vi "Simulator SNA Measure.vi"(8 "error in (no error)":errorcluster, 10 "SP Stimulus":T5={"Use Instrument Settings"=FALSE, "Blank Frequencies"=FALSE, "Sweep Type"=enum."Linear", "Sweep"={"Fstart"=500.0, "Fstop"=1500.0, "Units"=enum."MHz", "Points"=201}, "Power (dBm)"=999.0, "IFBW (Hz)"=-1.0, "Sweep Time (s)"=-1.0, "Calibration"={"State"=FALSE, "String"=""}} {"Sweep Time (s)" format="%.3g"}, 11 "Parameters to Measure":T1[](array[typedef]) {"Channel" min=1 max=99 step=1; "Parameter"."Stimulus Port" min=1 step=1; "Parameter"."Response Port" min=1 step=1}) -> (0 "error out":errorcluster, 2 "S Parameters":cluster{"f0":dbl, "df":dbl, cdb[][]}, 3 "Parameters to Measure":T1[](array[typedef]) {"Channel" min=1 max=99 step=1; "Parameter"."Stimulus Port" min=1 step=1; "Parameter"."Response Port" min=1 step=1})   [LabVIEW 2011]
uses:
  tests/S Parameter/TypeDefs/SP Stimulus Parameters.ctl
  tests/S Parameter/TypeDefs/SP Frequency Units.ctl
  tests/S Parameter/TypeDefs/SP Calibration State.ctl
  tests/S Parameter/TypeDefs/SP Parameter to Measure.ctl
  tests/S Parameter/TypeDefs/SP Parameter.ctl
  tests/S Parameter/TypeDefs/SP Measurement Format.ctl
panel:
  out "Plot S12":cluster{"f0":dbl, "df":dbl, dbl[][]}(graph)
  out "Plot S22":cluster{"Fstart, MHz":dbl, dbl, dbl[][]}(graph)
  out "Plot S21":cluster{"f0":dbl, "df":dbl, dbl[][]}(graph)
  out "Plot S11":cluster{"Fstart, MHz":dbl, dbl, dbl[][]}(graph)
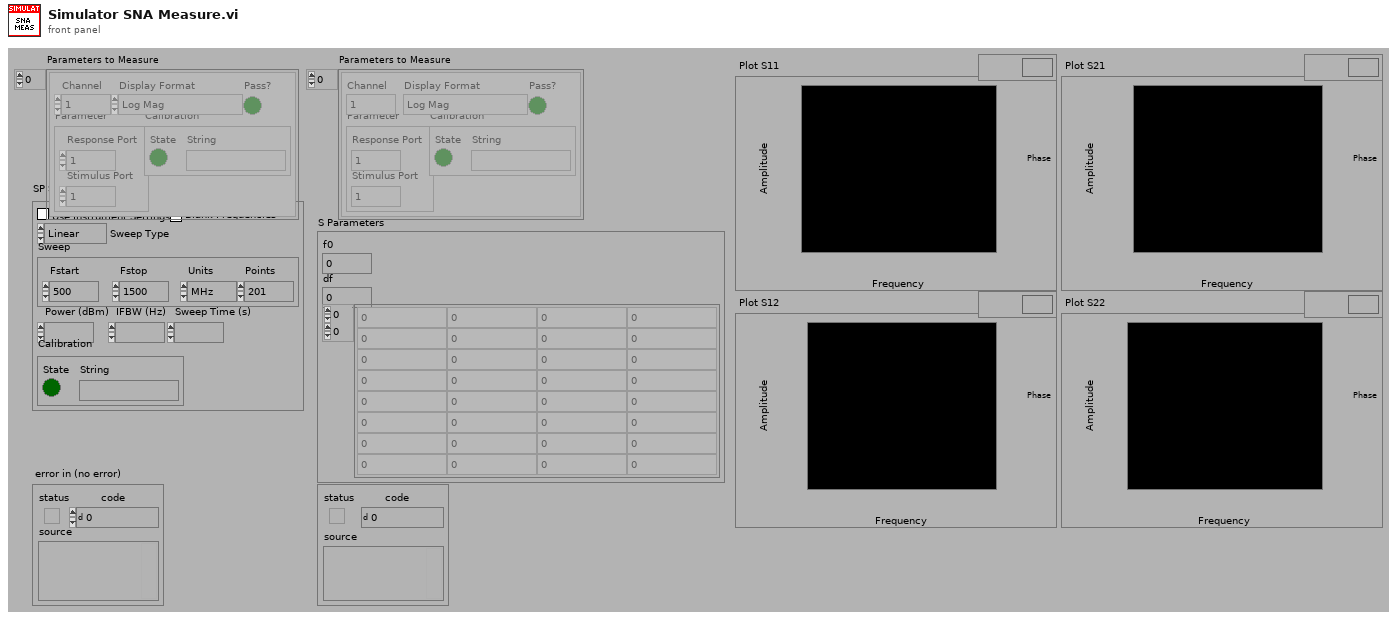
[diagram p1: front panel]
types:
  T1 = typedef "SP Parameter to Measure.ctl" = cluster{"Channel":i8, "Parameter":T2, "Calibration":T3, "Display Format":T4, "Pass?":bool}
  T2 = typedef "SP Parameter.ctl" = cluster{"Stimulus Port":i8, "Response Port":i8}
  T3 = typedef "SP Calibration State.ctl" = cluster{"State":bool, "String":string}
  T4 = typedef "SP Measurement Format.ctl" = enum32{"Log Mag", "Phase", "Delay", "Smith (R+jX)", "Polar (Re/Im)", "Linear Mag", "SWR", "Real", "Imaginary", "Smith (Lin/Phase)", "Smith (Log/Phase)", "Smith (Real/Imag)", "Smith (G+jB)", "Polar (Lin/Phase)", "Polar (Log/Phase)", "Expanded Phase", "Positive Phase", "Inverted Smith", "Unwrapped Phase", "Power Out", "Power In", "Linear Mag/Phase", "Log Mag/Phase", "Real/Imaginary"}
  T5 = typedef "SP Stimulus Parameters.ctl" = cluster{"Use Instrument Settings":bool, "Blank Frequencies":bool, "Sweep Type":enum32{"Linear", "Logarithmic", "List", "Power", "CW"}, "Sweep":cluster{"Fstart":dbl, "Fstop":dbl, "Units":T6, "Points":i32}, "Power (dBm)":dbl, "IFBW (Hz)":dbl, "Sweep Time (s)":dbl, "Calibration":T3}
  T6 = typedef "SP Frequency Units.ctl" = enum16{"Hz", "kHz", "MHz", "GHz", "Points"}
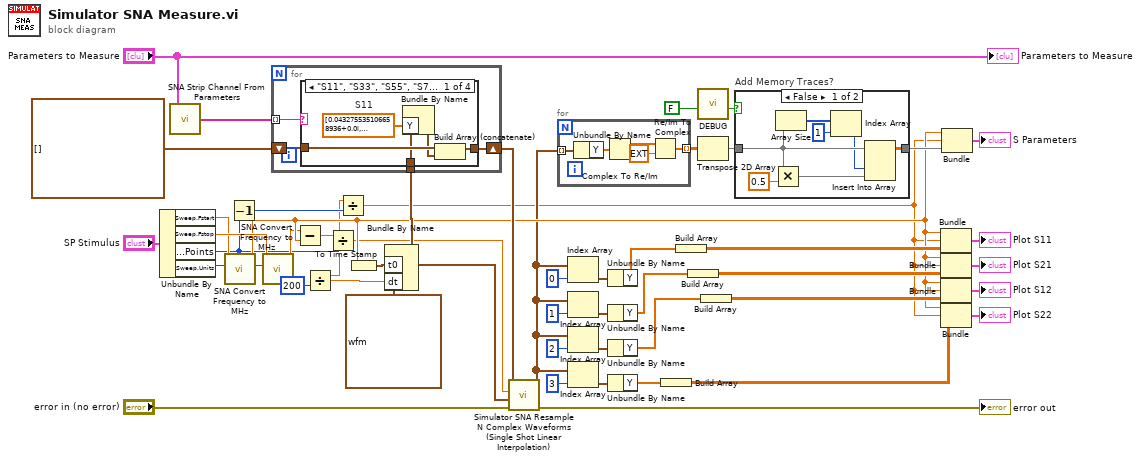
[diagram p0: block diagram]
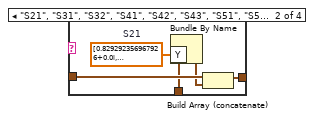
[diagram p3: hidden frame]
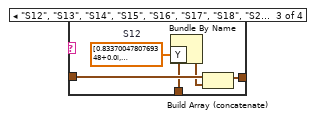
[diagram p4: hidden frame]
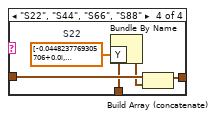
[diagram p5: hidden frame]
diagram:
  n1 = Unbundle By Name("SP Stimulus") -> ("Sweep.Fstart"=w11:dbl, "Sweep.Fstop"=w12:dbl, "Sweep.Points"=w4:i32, "Sweep.Units"=w8:T6)
  n2 = call "SNA Strip Channel From Parameters.vi"("Parameters to Measure"="Parameters to Measure") -> ("Parameters to Measure"=w47:string[])  [unwired: 4 out]
  n3 = call "SNA Convert Frequency to MHz.vi"("Units"=w8, "Frequency"=w11) -> ("Converted Frequency"=w10:dbl)  [unwired: 9 out]
  n4 = Decrement(x=w4) -> (x-1=w5:i32)
  n5 = call "SNA Convert Frequency to MHz.vi"("Units"=w8, "Frequency"=w12) -> ("Converted Frequency"=w9:dbl)  [unwired: 9 out]
  n6 = Subtract(x=w9, y=w10) -> (x-y=w3:dbl)
  n7 = Divide(x=w3, y=200 ("Points")) -> (x/y=w27:dbl)
  n8 = Divide(x=w3, y=w4) -> (x/y=w2:dbl)
  n9 = Divide(x=w3, y=w5) -> (x/y=w1:dbl)
  n10 = To Time Stamp(1:w10) -> (0:w26:timestamp)
  n11 = Bundle By Name(cluster=waveform(cdb) {"t0"=timestamp(0 s since 1904-01-01), "dt"=1.0, "Y"=[]} ("output waveform"), "t0"=w26, "dt"=w27) -> (w31:waveform(cdb))
  n12 = for {
    tunnel: w47 -> [w51] mode=indexing
    shift-right: [w52] -> w29
    shift-left: waveform(cdb)[] [] -> [w53]
    tunnel: w31 -> [w50]
    n13 = case shown="\"S11\", \"S33\", \"S55\", \"S77\", Default" w51 {
      tunnel: w53 -> [w58 w63 w68 w73]
      tunnel: [w57 w62 w67 w72] -> w52
      tunnel: w50 -> [w56 w61 w66 w71]
      frame "S11", "S33", "S55", "S77", Default {
        w55 = cdb[] [0.043275535106658936+0.0i, 0.039342574775218964+0.0i, 0.03575783222913742+0.0i, 0.032080549746751785+0.0i, 0.028698638081550598+0.0i, 0.025614049285650253+0.0i, 0.02282632142305374+0.0i, 0.020214837044477463+0.0i, 0.018059048801660538+0.0i, 0.015805359929800034+0.0i, 0.014122397638857365+0.0i, 0.012394579127430916+0.0i, 0.010067702271044254+0.0i, 0.008520152419805527+0.0i, 0.007258761674165726+0.0i, 0.005761267151683569+0.0i, 0.00486418791115284+0.0i, 0.0033858772367239+0.0i, 0.002761210547760129+0.0i, 0.0017304427456110716+0.0i, 0.0012977475998923182+0.0i, 0.0004616621881723404+0.0i, -1.719485044304747e-05+0.0i, -0.00042151467641815543+0.0i, -0.0007105278200469911+0.0i, -0.0012685193214565516+0.0i, -0.0019677081145346165+0.0i, -0.0026351099368184805+0.0i, -0.0033787309657782316+0.0i, -0.004169062245637178+0.0i, -0.004505419172346592+0.0i, -0.00413671275600791+0.0i, -0.0035033696331083775+0.0i, -0.003271963680163026+0.0i, -0.003496718592941761+0.0i, -0.003873205743730068+0.0i, -0.003999741747975349+0.0i, -0.003930048085749149+0.0i, -0.003324817167595029+0.0i, -0.0031607337296009064+0.0i, -0.0030308200512081385+0.0i, -0.0034498628228902817+0.0i, -0.003611180931329727+0.0i, -0.0037343313451856375+0.0i, -0.002879899460822344+0.0i, -0.002135245129466057+0.0i, -0.001469879411160946+0.0i, -0.0009730787132866681+0.0i, -0.0011905874125659466+0.0i, -0.0010869997786357999+0.0i, -0.0010538013884797692+0.0i, -0.000801632646471262+0.0i, -0.0003287283470854163+0.0i, -0.00020402256632223725+0.0i, -0.0002642142935656011+0.0i, -0.00013643794227391481+0.0i, 0.0005306923994794488+0.0i, 0.0014401909429579973+0.0i, 0.002155429683625698+0.0i, 0.0026408841367810965+0.0i, 0.002987817395478487+0.0i, 0.0032288457732647657+0.0i, 0.00361762847751379+0.0i, 0.0037104820366948843+0.0i, 0.004260951653122902+0.0i, 0.0044131227768957615+0.0i, 0.005049579311162233+0.0i, 0.0053521208465099335+0.0i, 0.006191197317093611+0.0i, 0.00685926852747798+0.0i, 0.007911991328001022+0.0i, 0.008351437747478485+0.0i, 0.008801144547760487+0.0i, 0.008953887969255447+0.0i, 0.009607013314962387+0.0i, 0.010086072608828545+0.0i, 0.010762657038867474+0.0i, 0.011188128031790257+0.0i, 0.011861111968755722+0.0i, 0.012636076658964157+0.0i, 0.01329171285033226+0.0i, 0.01419072039425373+0.0i, 0.014360726810991764+0.0i, 0.014936965890228748+0.0i, 0.014871757477521896+0.0i, 0.015183527953922749+0.0i, 0.015605935826897621+0.0i, 0.015983808785676956+0.0i, 0.01635676436126232+0.0i, 0.0168494563549757+0.0i, 0.01760626956820488+0.0i, 0.018216129392385483+0.0i, 0.018974874168634415+0.0i, 0.019734209403395653+0.0i, 0.01982462778687477+0.0i, 0.02016322687268257+0.0i, 0.02022622525691986+0.0i, 0.020693926140666008+0.0i, 0.020658815279603004+0.0i, 0.021412502974271774+0.0i, 0.021840233355760574+0.0i, 0.02223920449614525+0.0i, 0.022984003648161888+0.0i, 0.023274244740605354+0.0i, 0.0235948096960783+0.0i, 0.023692430928349495+0.0i, 0.023691050708293915+0.0i, 0.023721178993582726+0.0i, 0.023409923538565636+0.0i, 0.02332262136042118+0.0i, 0.0232867244631052+0.0i, 0.023343225941061974+0.0i, 0.02331232838332653+0.0i, 0.023639868944883347+0.0i, 0.023666899651288986+0.0i, 0.023931000381708145+0.0i, 0.024006182327866554+0.0i, 0.024024013429880142+0.0i, 0.02399740368127823+0.0i, 0.02352958731353283+0.0i, 0.02293366566300392+0.0i, 0.022277450188994408+0.0i, 0.02165168710052967+0.0i, 0.021030226722359657+0.0i, 0.020597459748387337+0.0i, 0.019762272015213966+0.0i, 0.01981099136173725+0.0i, 0.0190260112285614+0.0i, 0.01884141005575657+0.0i, 0.018474403768777847+0.0i, 0.018153464421629906+0.0i, 0.017230894416570663+0.0i, 0.01683255285024643+0.0i, 0.015972070395946503+0.0i, 0.014567862264811993+0.0i, 0.013760950416326523+0.0i, 0.012620450928807259+0.0i, 0.010907035320997238+0.0i, 0.009974002838134766+0.0i, 0.00895930826663971+0.0i, 0.007833925075829029+0.0i, 0.007271322887390852+0.0i, 0.006285695359110832+0.0i, 0.005394641775637865+0.0i, 0.004059544298797846+0.0i, 0.002686774358153343+0.0i, 0.0017567717004567385+0.0i, 0.0006243944517336786+0.0i, -0.0004936228506267071+0.0i, -0.0028370742220431566+0.0i, -0.005315746646374464+0.0i, -0.0071689714677631855+0.0i, -0.007896475493907928+0.0i, -0.008393912576138973+0.0i, -0.009499276988208294+0.0i, -0.010864137671887875+0.0i, -0.013279550708830357+0.0i, -0.015229152515530586+0.0i, -0.016355840489268303+0.0i, -0.01756197027862072+0.0i, -0.018781857565045357+0.0i, -0.021512817591428757+0.0i, -0.025313854217529297+0.0i, -0.027553554624319077+0.0i, -0.028660070151090622+0.0i, -0.028027910739183426+0.0i, -0.02755579724907875+0.0i, -0.028688842430710793+0.0i, -0.03104601986706257+0.0i, -0.03363754600286484+0.0i, -0.03597893938422203+0.0i, -0.03675049543380737+0.0i, -0.03752102330327034+0.0i, -0.03978640213608742+0.0i, -0.042819179594516754+0.0i, -0.047085169702768326+0.0i, -0.049191735684871674+0.0i, -0.04951959848403931+0.0i, -0.04790704324841499+0.0i, -0.04758603125810623+0.0i, -0.04839025065302849+0.0i, -0.05057644844055176+0.0i, -0.0533347986638546+0.0i, -0.05488186329603195+0.0i, -0.05515661835670471+0.0i, -0.05508638545870781+0.0i, -0.055647045373916626+0.0i, -0.05629001185297966+0.0i, -0.05946866795420647+0.0i, -0.06072845682501793+0.0i, -0.06155878305435181+0.0i, -0.0606592521071434+0.0i, -0.060178909450769424+0.0i, -0.05885367840528488+0.0i, -0.06058591604232788+0.0i, -0.06147431954741478+0.0i, -0.06279278546571732+0.0i, -0.06465675681829453+0.0i, -0.06480240076780319+0.0i, -0.06487281620502472+0.0i, -0.06429072469472885+0.0i]  # S11
        n14 = Bundle By Name(cluster=w56, "Y"=w55) -> (w54:waveform(cdb))
        n15 = Build Array (concatenate)(w58, w54) -> (w57:waveform(cdb)[])
      }
      frame "S21", "S31", "S32", "S41", "S42", "S43", "S51", "S52", "S53", "S54", "S61", "S62", "S63", "S64", "S65", "S71", "S72", "S73", "S74", "S75", "S76", "S81", "S82", "S83", "S84", "S85", "S86", "S87" {
        w59 = cdb[] [0.829292356967926+0.0i, 0.814454197883606+0.0i, 0.7981213331222534+0.0i, 0.7870112657546997+0.0i, 0.7711793184280396+0.0i, 0.7556583285331726+0.0i, 0.7388772964477539+0.0i, 0.7228282690048218+0.0i, 0.7071607112884521+0.0i, 0.6912792325019836+0.0i, 0.6753528118133545+0.0i, 0.6560407876968384+0.0i, 0.6371591091156006+0.0i, 0.6180185079574585+0.0i, 0.6032703518867493+0.0i, 0.5853940844535828+0.0i, 0.5672386288642883+0.0i, 0.5465737581253052+0.0i, 0.5287693738937378+0.0i, 0.5108529925346375+0.0i, 0.4929536283016205+0.0i, 0.4726460576057434+0.0i, 0.45388948917388916+0.0i, 0.4329501986503601+0.0i, 0.41499051451683044+0.0i, 0.3953711688518524+0.0i, 0.37639090418815613+0.0i, 0.35440051555633545+0.0i, 0.3362242579460144+0.0i, 0.31509923934936523+0.0i, 0.29575711488723755+0.0i, 0.2755361497402191+0.0i, 0.2568615674972534+0.0i, 0.23595577478408813+0.0i, 0.21444492042064667+0.0i, 0.19693320989608765+0.0i, 0.17813338339328766+0.0i, 0.15588150918483734+0.0i, 0.13776037096977234+0.0i, 0.11660043895244598+0.0i, 0.09747599810361862+0.0i, 0.07880620658397675+0.0i, 0.05615612864494324+0.0i, 0.0381329171359539+0.0i, 0.016294067725539207+0.0i, -0.003492713673040271+0.0i, -0.021831337362527847+0.0i, -0.0421501062810421+0.0i, -0.061345260590314865+0.0i, -0.08185604959726334+0.0i, -0.09892823547124863+0.0i, -0.12116867303848267+0.0i, -0.1380733698606491+0.0i, -0.15851135551929474+0.0i, -0.1788916140794754+0.0i, -0.19643454253673553+0.0i, -0.21329368650913239+0.0i, -0.2337159663438797+0.0i, -0.25253576040267944+0.0i, -0.270393967628479+0.0i, -0.2902970314025879+0.0i, -0.3075717091560364+0.0i, -0.32540351152420044+0.0i, -0.3427804410457611+0.0i, -0.358801931142807+0.0i, -0.3782116174697876+0.0i, -0.3964827358722687+0.0i, -0.4130129814147949+0.0i, -0.42976996302604675+0.0i, -0.44708988070487976+0.0i, -0.4636856019496918+0.0i, -0.48080843687057495+0.0i, -0.4962398409843445+0.0i, -0.5128710269927979+0.0i, -0.5280305743217468+0.0i, -0.5448092818260193+0.0i, -0.5582361817359924+0.0i, -0.5728786587715149+0.0i, -0.5888417363166809+0.0i, -0.6064391136169434+0.0i, -0.6201893091201782+0.0i, -0.6338473558425903+0.0i, -0.6467384696006775+0.0i, -0.6618889570236206+0.0i, -0.676064670085907+0.0i, -0.6866525411605835+0.0i, -0.7018538117408752+0.0i, -0.7150512337684631+0.0i, -0.728316068649292+0.0i, -0.7392727136611938+0.0i, -0.7518630027770996+0.0i, -0.7645359635353088+0.0i, -0.7738081812858582+0.0i, -0.7883812189102173+0.0i, -0.7997139096260071+0.0i, -0.8098510503768921+0.0i, -0.8207243084907532+0.0i, -0.8297194838523865+0.0i, -0.8402549028396606+0.0i, -0.8492640852928162+0.0i, -0.8584194183349609+0.0i, -0.8675045371055603+0.0i, -0.873566210269928+0.0i, -0.8841186761856079+0.0i, -0.8934317827224731+0.0i, -0.9010100960731506+0.0i, -0.9081630110740662+0.0i, -0.9165226817131042+0.0i, -0.921902060508728+0.0i, -0.929990291595459+0.0i, -0.9349827766418457+0.0i, -0.9424318671226501+0.0i, -0.9459336996078491+0.0i, -0.9520758390426636+0.0i, -0.9587121605873108+0.0i, -0.9634407162666321+0.0i, -0.9670430421829224+0.0i, -0.9712170362472534+0.0i, -0.9760630130767822+0.0i, -0.9790180325508118+0.0i, -0.9799625277519226+0.0i, -0.9845265746116638+0.0i, -0.987425684928894+0.0i, -0.989444375038147+0.0i, -0.9929931163787842+0.0i, -0.9935646057128906+0.0i, -0.9969585537910461+0.0i, -0.9946895837783813+0.0i, -0.9962232708930969+0.0i, -0.9964486360549927+0.0i, -0.9962095022201538+0.0i, -0.996056318283081+0.0i, -0.9940896034240723+0.0i, -0.9956469535827637+0.0i, -0.9917272329330444+0.0i, -0.9910922646522522+0.0i, -0.9918628334999084+0.0i, -0.986739456653595+0.0i, -0.9865198731422424+0.0i, -0.9832531809806824+0.0i, -0.980251669883728+0.0i, -0.9778366088867188+0.0i, -0.972420334815979+0.0i, -0.9679995179176331+0.0i, -0.9628635048866272+0.0i, -0.9585220813751221+0.0i, -0.9528169631958008+0.0i, -0.9470780491828918+0.0i, -0.9426121711730957+0.0i, -0.9383622407913208+0.0i, -0.9331514835357666+0.0i, -0.9263299703598022+0.0i, -0.9203755259513855+0.0i, -0.913105309009552+0.0i, -0.9034777283668518+0.0i, -0.8951209187507629+0.0i, -0.8883877992630005+0.0i, -0.879611074924469+0.0i, -0.8694924712181091+0.0i, -0.8617876768112183+0.0i, -0.853515088558197+0.0i, -0.8449181318283081+0.0i, -0.8350080251693726+0.0i, -0.8312739729881287+0.0i, -0.8206787109375+0.0i, -0.8102623820304871+0.0i, -0.7970291376113892+0.0i, -0.7831966876983643+0.0i, -0.7730605602264404+0.0i, -0.7591240406036377+0.0i, -0.7464131116867065+0.0i, -0.7364375591278076+0.0i, -0.7251046299934387+0.0i, -0.7161509394645691+0.0i, -0.7067240476608276+0.0i, -0.6938031315803528+0.0i, -0.6799384355545044+0.0i, -0.6680499315261841+0.0i, -0.6545169353485107+0.0i, -0.6385235786437988+0.0i, -0.6245161294937134+0.0i, -0.6076085567474365+0.0i, -0.5907292366027832+0.0i, -0.5797586441040039+0.0i, -0.5657033920288086+0.0i, -0.5516921877861023+0.0i, -0.5354703664779663+0.0i, -0.523349404335022+0.0i, -0.5107196569442749+0.0i, -0.49576160311698914+0.0i, -0.48084160685539246+0.0i, -0.4637007713317871+0.0i, -0.44816768169403076+0.0i, -0.42999717593193054+0.0i, -0.413239449262619+0.0i, -0.3964954614639282+0.0i, -0.37846991419792175+0.0i, -0.36190730333328247+0.0i, -0.3453793525695801+0.0i, -0.32939761877059937+0.0i, -0.31479111313819885+0.0i]  # S21
        n16 = Bundle By Name(cluster=w61, "Y"=w59) -> (w60:waveform(cdb))
        n17 = Build Array (concatenate)(w63, w60) -> (w62:waveform(cdb)[])
      }
      frame "S12", "S13", "S14", "S15", "S16", "S17", "S18", "S23", "S24", "S25", "S26", "S27", "S28", "S34", "S35", "S36", "S37", "S38", "S45", "S46", "S47", "S48", "S56", "S57", "S58", "S67", "S68", "S78" {
        w64 = cdb[] [0.8337004780769348+0.0i, 0.8181808590888977+0.0i, 0.8031412959098816+0.0i, 0.7909902334213257+0.0i, 0.7788154482841492+0.0i, 0.7681070566177368+0.0i, 0.7551140785217285+0.0i, 0.7417704463005066+0.0i, 0.7248368859291077+0.0i, 0.7070673704147339+0.0i, 0.6861556768417358+0.0i, 0.6654462218284607+0.0i, 0.637874960899353+0.0i, 0.6171132922172546+0.0i, 0.5911676287651062+0.0i, 0.5713427066802979+0.0i, 0.5516795516014099+0.0i, 0.5347855091094971+0.0i, 0.5204638242721558+0.0i, 0.5077767372131348+0.0i, 0.4974057078361511+0.0i, 0.4838629364967346+0.0i, 0.46762534976005554+0.0i, 0.4514274597167969+0.0i, 0.4292939007282257+0.0i, 0.40243837237358093+0.0i, 0.37349605560302734+0.0i, 0.34189796447753906+0.0i, 0.3098517060279846+0.0i, 0.2839166820049286+0.0i, 0.2591840326786041+0.0i, 0.24050498008728027+0.0i, 0.2294185906648636+0.0i, 0.2192041575908661+0.0i, 0.21159739792346954+0.0i, 0.2037205696105957+0.0i, 0.19587396085262299+0.0i, 0.17845891416072845+0.0i, 0.15374864637851715+0.0i, 0.12296313047409058+0.0i, 0.08836781978607178+0.0i, 0.05404189974069595+0.0i, 0.021986862644553185+0.0i, -0.00695606367662549+0.0i, -0.028587350621819496+0.0i, -0.04182153567671776+0.0i, -0.05166104435920715+0.0i, -0.05838768184185028+0.0i, -0.06793583929538727+0.0i, -0.07563966512680054+0.0i, -0.09253257513046265+0.0i, -0.11477933824062347+0.0i, -0.13989581167697906+0.0i, -0.17279675602912903+0.0i, -0.20106659829616547+0.0i, -0.22970663011074066+0.0i, -0.25439924001693726+0.0i, -0.2693353295326233+0.0i, -0.2889915406703949+0.0i, -0.29486438632011414+0.0i, -0.3078099489212036+0.0i, -0.32018768787384033+0.0i, -0.33861541748046875+0.0i, -0.3564850091934204+0.0i, -0.3752939999103546+0.0i, -0.3948507308959961+0.0i, -0.41648608446121216+0.0i, -0.43723639845848083+0.0i, -0.452502578496933+0.0i, -0.46733251214027405+0.0i, -0.48071280121803284+0.0i, -0.49225661158561707+0.0i, -0.506791889667511+0.0i, -0.5197045803070068+0.0i, -0.5357764363288879+0.0i, -0.5509658455848694+0.0i, -0.5691072344779968+0.0i, -0.5897894501686096+0.0i, -0.605778157711029+0.0i, -0.6210479140281677+0.0i, -0.6325191855430603+0.0i, -0.6439656615257263+0.0i, -0.6548815965652466+0.0i, -0.6662686467170715+0.0i, -0.6743442416191101+0.0i, -0.6855710744857788+0.0i, -0.7000376582145691+0.0i, -0.7117102146148682+0.0i, -0.7253685593605042+0.0i, -0.7386612296104431+0.0i, -0.7532441020011902+0.0i, -0.765815794467926+0.0i, -0.7768866419792175+0.0i, -0.7853107452392578+0.0i, -0.7932745218276978+0.0i, -0.800614058971405+0.0i, -0.8092449903488159+0.0i, -0.8147201538085938+0.0i, -0.8231639862060547+0.0i, -0.830460250377655+0.0i, -0.8419719338417053+0.0i, -0.8522282838821411+0.0i, -0.8624382019042969+0.0i, -0.8695622086524963+0.0i, -0.8771089315414429+0.0i, -0.8840516209602356+0.0i, -0.888999342918396+0.0i, -0.891585111618042+0.0i, -0.8962506055831909+0.0i, -0.9008564949035645+0.0i, -0.9058078527450562+0.0i, -0.913115382194519+0.0i, -0.9204257130622864+0.0i, -0.9283400774002075+0.0i, -0.935961902141571+0.0i, -0.9418730735778809+0.0i, -0.9456731081008911+0.0i, -0.9482985734939575+0.0i, -0.9491007924079895+0.0i, -0.9507501721382141+0.0i, -0.9520665407180786+0.0i, -0.9530963897705078+0.0i, -0.9568275213241577+0.0i, -0.9600855112075806+0.0i, -0.9627634882926941+0.0i, -0.9671722650527954+0.0i, -0.9694264531135559+0.0i, -0.971646249294281+0.0i, -0.972331702709198+0.0i, -0.9724413156509399+0.0i, -0.9702968597412109+0.0i, -0.9721423983573914+0.0i, -0.9718196392059326+0.0i, -0.9726036190986633+0.0i, -0.9727047681808472+0.0i, -0.9739677309989929+0.0i, -0.9713402986526489+0.0i, -0.9660041332244873+0.0i, -0.960610032081604+0.0i, -0.956613302230835+0.0i, -0.9506188035011292+0.0i, -0.948957622051239+0.0i, -0.9482381939888+0.0i, -0.9498124122619629+0.0i, -0.9518067240715027+0.0i, -0.9508785605430603+0.0i, -0.9477074146270752+0.0i, -0.9427552819252014+0.0i, -0.9327554702758789+0.0i, -0.9165830612182617+0.0i, -0.9024083018302917+0.0i, -0.891497790813446+0.0i, -0.8820448517799377+0.0i, -0.8806410431861877+0.0i, -0.8812286257743835+0.0i, -0.88673335313797+0.0i, -0.8888771533966064+0.0i, -0.8925393223762512+0.0i, -0.8883774876594543+0.0i, -0.8752503395080566+0.0i, -0.8541203737258911+0.0i, -0.8287928104400635+0.0i, -0.7984622716903687+0.0i, -0.7784661054611206+0.0i, -0.7642708420753479+0.0i, -0.7597957253456116+0.0i, -0.7634502649307251+0.0i, -0.7701605558395386+0.0i, -0.777458131313324+0.0i, -0.7836854457855225+0.0i, -0.781994640827179+0.0i, -0.7683941125869751+0.0i, -0.7450302839279175+0.0i, -0.7109066247940063+0.0i, -0.6751865148544312+0.0i, -0.6423426270484924+0.0i, -0.6172760128974915+0.0i, -0.6061503291130066+0.0i, -0.6009782552719116+0.0i, -0.6047084927558899+0.0i, -0.613054096698761+0.0i, -0.6205593943595886+0.0i, -0.6221399307250977+0.0i, -0.618950366973877+0.0i, -0.6042948365211487+0.0i, -0.5778829455375671+0.0i, -0.5433223843574524+0.0i, -0.509933352470398+0.0i, -0.4719630777835846+0.0i, -0.4437721371650696+0.0i, -0.4217017590999603+0.0i, -0.4115893244743347+0.0i, -0.4102535843849182+0.0i, -0.4117880165576935+0.0i, -0.4139910340309143+0.0i, -0.4183366298675537+0.0i, -0.4167386591434479+0.0i, -0.4066200256347656+0.0i, -0.38806724548339844+0.0i, -0.3580075204372406+0.0i, -0.3183501064777374+0.0i]  # S12
        n18 = Bundle By Name(cluster=w66, "Y"=w64) -> (w65:waveform(cdb))
        n19 = Build Array (concatenate)(w68, w65) -> (w67:waveform(cdb)[])
      }
      frame "S22", "S44", "S66", "S88" {
        w69 = cdb[] [-0.0448237769305706+0.0i, -0.04102639853954315+0.0i, -0.03737544268369675+0.0i, -0.034089814871549606+0.0i, -0.030959470197558403+0.0i, -0.028162462636828423+0.0i, -0.02541796676814556+0.0i, -0.023308314383029938+0.0i, -0.02091742493212223+0.0i, -0.018918225541710854+0.0i, -0.017081458121538162+0.0i, -0.015482684597373009+0.0i, -0.014000953175127506+0.0i, -0.01254727877676487+0.0i, -0.011165780946612358+0.0i, -0.010345423594117165+0.0i, -0.009379100054502487+0.0i, -0.00840721745043993+0.0i, -0.007564597763121128+0.0i, -0.006762946490198374+0.0i, -0.0059876772575080395+0.0i, -0.005517164245247841+0.0i, -0.004945616703480482+0.0i, -0.004484861623495817+0.0i, -0.004106960259377956+0.0i, -0.0040862238965928555+0.0i, -0.004174944944679737+0.0i, -0.003841354977339506+0.0i, -0.004038045182824135+0.0i, -0.0041593159548938274+0.0i, -0.0044232625514268875+0.0i, -0.0041390941478312016+0.0i, -0.004399512894451618+0.0i, -0.004216721281409264+0.0i, -0.004327621776610613+0.0i, -0.004233787301927805+0.0i, -0.004186590202152729+0.0i, -0.004376720171421766+0.0i, -0.004460547119379044+0.0i, -0.004746682476252317+0.0i, -0.005126139149069786+0.0i, -0.00522314989939332+0.0i, -0.005602819379419088+0.0i, -0.005595334339886904+0.0i, -0.005792031995952129+0.0i, -0.005758288316428661+0.0i, -0.005966282915323973+0.0i, -0.005686081945896149+0.0i, -0.005799978971481323+0.0i, -0.005790566559880972+0.0i, -0.006069929338991642+0.0i, -0.006077638361603022+0.0i, -0.006143453996628523+0.0i, -0.006082667037844658+0.0i, -0.006236350629478693+0.0i, -0.006148894317448139+0.0i, -0.006158811971545219+0.0i, -0.005938847549259663+0.0i, -0.005814449395984411+0.0i, -0.005655704066157341+0.0i, -0.005622300785034895+0.0i, -0.005354489199817181+0.0i, -0.005245627369731665+0.0i, -0.005094286985695362+0.0i, -0.005099698435515165+0.0i, -0.0047679501585662365+0.0i, -0.004622514359652996+0.0i, -0.004251937381923199+0.0i, -0.004076929297298193+0.0i, -0.0038552219048142433+0.0i, -0.0036175204440951347+0.0i, -0.0032895402982831+0.0i, -0.0030748452991247177+0.0i, -0.0027343553956598043+0.0i, -0.0026735644787549973+0.0i, -0.0024386083241552114+0.0i, -0.0022648742888122797+0.0i, -0.0021435734815895557+0.0i, -0.0020642667077481747+0.0i, -0.0019470123806968331+0.0i, -0.0016891410341486335+0.0i, -0.001467305002734065+0.0i, -0.001399420783855021+0.0i, -0.0010558502981439233+0.0i, -0.0008833135943859816+0.0i, -0.000758141977712512+0.0i, -0.00048745161620900035+0.0i, -0.0003483314940240234+0.0i, -0.00028839983860962093+0.0i, -6.241415394470096e-05+0.0i, 5.908060848014429e-05+0.0i, 0.00019588899158407003+0.0i, 0.00027953420067206025+0.0i, 0.00035175096127204597+0.0i, 0.0003388347977306694+0.0i, 0.00045757752377539873+0.0i, 0.0004954376490786672+0.0i, 0.0004994297050870955+0.0i, 0.0004787541402038187+0.0i, 0.0004915528697893023+0.0i, 0.0004942804225720465+0.0i, 0.0004837051674257964+0.0i, 0.0004830575198866427+0.0i, 0.00048056108062155545+0.0i, 0.0004647464957088232+0.0i, 0.00045925183803774416+0.0i, 0.00039012142224237323+0.0i, 0.00036192749394103885+0.0i, 0.0003474172262940556+0.0i, 0.0003007917548529804+0.0i, 0.0002585411712061614+0.0i, 0.00020978024986106902+0.0i, 9.311280882684514e-05+0.0i, 3.437729537836276e-05+0.0i, -2.6182860892731696e-05+0.0i, -9.559790487401187e-05+0.0i, -0.00012796329974662513+0.0i, -0.00016629937454126775+0.0i, -0.00018859354895539582+0.0i, -0.00016769948706496507+0.0i, -0.00018103173351846635+0.0i, -0.00018724691472016275+0.0i, -0.0001743300526868552+0.0i, -0.0001649048354011029+0.0i, -0.00015603502106387168+0.0i, -0.00013644371938426048+0.0i, -9.474530816078186e-05+0.0i, -5.9985057305311784e-05+0.0i, 8.870118108461611e-06+0.0i, 9.934559784596786e-05+0.0i, 0.00018127325165551156+0.0i, 0.0002790482831187546+0.0i, 0.00038650145870633423+0.0i, 0.000505543255712837+0.0i, 0.0006492372485809028+0.0i, 0.000811923120636493+0.0i, 0.0009885950712487102+0.0i, 0.001171267475001514+0.0i, 0.001365330652333796+0.0i, 0.0015696100890636444+0.0i, 0.0017706482904031873+0.0i, 0.0019801591988652945+0.0i, 0.002092361217364669+0.0i, 0.0023044664412736893+0.0i, 0.0025349468924105167+0.0i, 0.002791930455714464+0.0i, 0.0030656736344099045+0.0i, 0.0033251012209802866+0.0i, 0.0036497320979833603+0.0i, 0.003974618390202522+0.0i, 0.004179029725492001+0.0i, 0.004448150750249624+0.0i, 0.004605614580214024+0.0i, 0.004715103656053543+0.0i, 0.004872438497841358+0.0i, 0.005027373321354389+0.0i, 0.005337926093488932+0.0i, 0.005487888585776091+0.0i, 0.005758954677730799+0.0i, 0.005848472472280264+0.0i, 0.006054707802832127+0.0i, 0.006243602838367224+0.0i, 0.006152447313070297+0.0i, 0.006166351027786732+0.0i, 0.006093923468142748+0.0i, 0.005887094419449568+0.0i, 0.0057772016152739525+0.0i, 0.005688414443284273+0.0i, 0.005684699863195419+0.0i, 0.005622982047498226+0.0i, 0.005431497003883123+0.0i, 0.005171825643628836+0.0i, 0.004884790629148483+0.0i, 0.004366884473711252+0.0i, 0.003925090655684471+0.0i, 0.003188987961038947+0.0i, 0.0027057796251028776+0.0i, 0.0021417015232145786+0.0i, 0.0015629694098606706+0.0i, 0.0010502667864784598+0.0i, 0.0004264943127054721+0.0i, -7.472128345398232e-05+0.0i, -0.0008630462107248604+0.0i, -0.001326490775682032+0.0i, -0.002498344052582979+0.0i, -0.003656521439552307+0.0i, -0.005031170789152384+0.0i, -0.006442666053771973+0.0i, -0.007896801456809044+0.0i, -0.009163213893771172+0.0i, -0.010341767221689224+0.0i, -0.011778250336647034+0.0i, -0.012648561969399452+0.0i, -0.013558346778154373+0.0i, -0.014745736494660378+0.0i, -0.016558662056922913+0.0i, -0.017478901892900467+0.0i, -0.019446969032287598+0.0i, -0.0211798045784235+0.0i, -0.023336362093687057+0.0i, -0.025581542402505875+0.0i]  # S22
        n20 = Bundle By Name(cluster=w71, "Y"=w69) -> (w70:waveform(cdb))
        n21 = Build Array (concatenate)(w73, w70) -> (w72:waveform(cdb)[])
      }
    }
  }
  n22 = call "Simulator SNA Resample N Complex Waveforms (Single Shot Linear Interpolation).vi"("error in (no error)"="error in (no error)", "t0"=w26, "dt"=w2, "waveforms in"=w29) -> ("error out"=→"error out":errorcluster, "resampled waveforms out"=w7:waveform(cdb)[])  [unwired: 1 in, 5 out]
  n23 = for {
    tunnel: w7 -> [w78] mode=indexing
    tunnel: [w74] -> w6 mode=indexing
    n24 = Unbundle By Name(w78) -> ("Y"=w75:cdb[])
    n25 = Complex To Re/Im(x + iy=w75) -> (x=w76:dbl[])  [unwired: 1 out]
    n26 = Re/Im To Complex(1:ext 0.0 ("y"), 2:w76) -> (0:w74:cxt[])
  }
  n27 = Index Array(array=w7, index=0 ("disabled index (col)")) -> (element=w20:waveform(cdb))
  n28 = Index Array(array=w7, index=1 ("disabled index (col)")) -> (element=w19:waveform(cdb))
  n29 = Index Array(array=w7, index=2 ("disabled index (col)")) -> (element=w18:waveform(cdb))
  n30 = Index Array(array=w7, index=3 ("disabled index (col)")) -> (element=w21:waveform(cdb))
  n31 = Unbundle By Name(w20) -> ("Y"=w17:cdb[])
  n32 = Unbundle By Name(w19) -> ("Y"=w16:cdb[])
  n33 = Unbundle By Name(w18) -> ("Y"=w15:cdb[])
  n34 = Unbundle By Name(w21) -> ("Y"=w14:cdb[])
  n35 = Build Array(w14) -> (w41:cdb[][])
  n36 = Build Array(w17) -> (w38:cdb[][])
  n37 = Build Array(w16) -> (w39:cdb[][])
  n38 = call "DEBUG.vi"("Dev DEBUG? (f)"=FALSE) -> ("DEBUG?"=w43:bool)  [unwired: 1 in, 5 out]
  n39 = Transpose 2D Array(2D array=w6) -> (transposed array=w13:cxt[][])
  n40 = Build Array(w15) -> (w40:cdb[][])
  n41 = case "Add Memory Traces?" shown="False" w43 {
    tunnel: [w84 w86] -> w45
    tunnel: w13 -> [w83 w86]
    frame False {
      n42 = Multiply(x=w83, y=0.5) -> (x*y=w79:cxt[][])
      n43 = Array Size(array=w83) -> (size(s)=w82:i32[])
      n44 = Index Array(array=w82, index=1) -> (element=w80:i32)
      n45 = Insert Into Array(array=w83, index (col)=w80, new element=w79) -> (w84:cxt[][])  [unwired: 1 in]
    }
    frame True {
      # "Do not add memory traces."
    }
  }
  n46 = Bundle("Converted Frequency"=w10, w1, w38) -> (→"Plot S11":cluster{"Converted Frequency":dbl, dbl, cdb[][]})  [unwired: 1 out]
  n47 = Bundle("Converted Frequency"=w10, w1, w39) -> (→"Plot S21":cluster{"Converted Frequency":dbl, dbl, cdb[][]})  [unwired: 1 out]
  n48 = Bundle("Converted Frequency"=w10, w1, w40) -> (→"Plot S12":cluster{"Converted Frequency":dbl, dbl, cdb[][]})  [unwired: 1 out]
  n49 = Bundle("Converted Frequency"=w10, w1, w41) -> (→"Plot S22":cluster{"Converted Frequency":dbl, dbl, cdb[][]})  [unwired: 1 out]
  n50 = Bundle("Converted Frequency"=w10, w1, w45) -> (→"S Parameters":cluster{"Converted Frequency":dbl, dbl, cxt[][]})  [unwired: 1 out]
  "Parameters to Measure" <- "Parameters to Measure"
